vi "ToSTM.vi"(0 "Port":refnum<visa-resource-name>="COM6", 1 "Baud":u32=115200, 3 "write buffer":string) -> (17 "read buffer":string)   [LabVIEW 2020]
uses:
  <vilib>/Instr/_visa.llb/VISA Configure Serial Port (Instr).vi
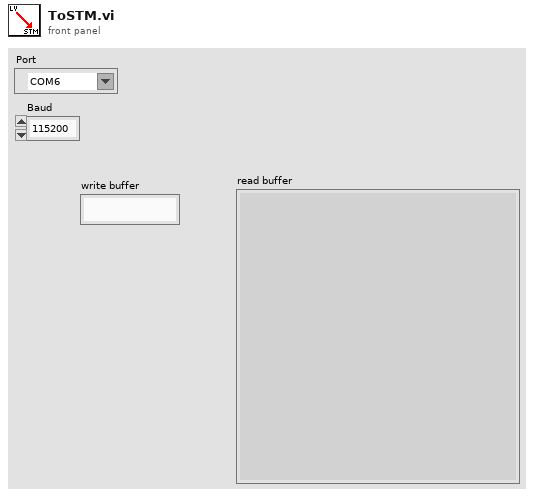
[diagram p1: front panel]
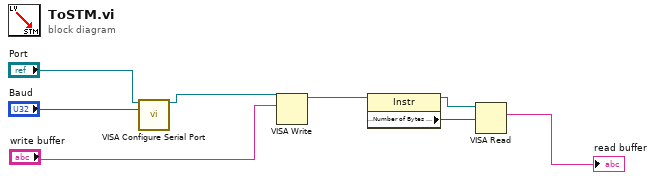
[diagram p0: block diagram]
diagram:
  n1 = call-poly "VISA Configure Serial Port"("VISA resource name"="Port", "baud rate (9600)"="Baud") -> ("VISA resource name out"=w5:refnum<visa-resource-name>)  [unwired: 12 in, 1 out]
  n2 = VISA Write(VISA resource name=w5, write buffer="write buffer") -> (VISA resource name out=w6:refnum<visa-resource-name>)  [unwired: 1 in, 2 out]
  n3 = property class="Instr"(reference=w6) -> (reference out=w7:refnum<visa-resource-name>, "Serial Settings:Number of Bytes at Serial Port"=w8:u32)  [unwired: 1 in, 1 out]
  n4 = VISA Read(VISA resource name=w7, byte count=w8) -> (read buffer=→"read buffer":string)  [unwired: 1 in, 3 out]
